vi "SineGen IP.vi"(7 "Reset Accumulator":bool, 9 "Signal Amplitude (x 2^15)":u16=32768, 10 "Phase Shift":u32, 11 "Accumulator Increment":u32=100000) -> (2 "Accumulator Value":u32 format="%.3e", 3 "Signal Value":i16)   [LabVIEW 2017]
doc: "This VI generates the next point on a DDS generated sine wave.\n\nThe accumulator increments to calculate the next phase value in the waveform. By varying the accumulator increment you control the frequency of the sine wave.\n\nThe accumulator phase value is used to select a value from the sine wave reference waveform stored in the Lookup Table VI. The waveformcan be p[hase shifted by specifying a non-zero phase shift value which is added to the accumulator phase. The output from the LUT is scaled using the AO Amplitude value."
uses:
  <vilib>/rvi/Arithmetic/AddSubMult/XNode/nirviSatArithmetic.xnode
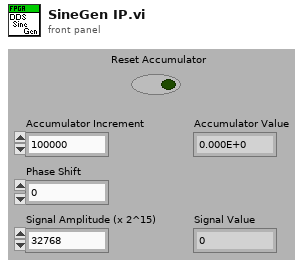
[diagram p1: front panel]
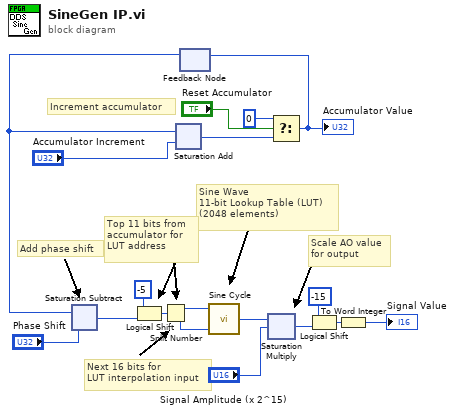
[diagram p0: block diagram]
diagram:
  # "Add phase shift"
  # "Increment accumulator"
  # "Scale AO value\nfor output"
  # "Next 16 bits for\nLUT interpolation input"
  # "Top 11 bits from \naccumulator for\nLUT address"
  # "Sine Wave \n11-bit Lookup Table (LUT)\n(2048 elements)"
  n1 = feedback #1() -> (w2:u32)  [unwired: 1 in]
  n2 = xnode "Saturation Subtract"("x"=w2, "y"="Phase Shift") -> ("x-y"=w1:u32)
  n3 = Logical Shift(y=-5, x=w1) -> (x << y=w11:u32)
  n4 = Split Number(x=w11) -> (hi(x)=w12:u16, lo(x)=w13:u16)
  n5 = xnode ("Saturation Add")("x"=w2, "y"="Accumulator Increment") -> ("x+y"=w8:u32)
  n6 = call "Sine Cycle"("address"=w12, "fractional index (x 2^16)"=w13) -> ("data out"=w14:i16)  [unwired: 7 in]
  n7 = xnode ("Saturation Multiply")("x"=w14, "y"="Signal Amplitude (x 2^15)") -> ("x*y"=w16:i32)
  n8 = Select(t=u32 0, s="Reset Accumulator", f=w8) -> (s? t:f=w10:u32)
  "Accumulator Value" <- w10
  n9 = feedback-in #1(w10) -> ()
  n10 = Logical Shift(y=-15, x=w16) -> (x << y=w18:i32)
  n11 = To Word Integer(number=w18) -> (16bit integer=→"Signal Value":i16)
